vi "TX_basic.vi"() -> ()   [LabVIEW 2019]
uses:
  <vilib>/sound2/lvsound2.llb/Sound File Info (path).vi
  <vilib>/sound2/lvsound2.llb/Sound File Read Open.vi
  <vilib>/Analysis/2dsp.llb/Rational Resample (single channel, DBL).vi
  <vilib>/express/express analysis/Spectral/Block/exnSpectralBlock spectral measurements RMS poly.vi
  <vilib>/express/express analysis/Spectral/Block/exnSpectralBlock spectral measurements RMS DDT.vi
  <instrlib>/niUSRP/niUSRP Write Tx Data (CDB).vi
  <vilib>/sound2/lvsound2.llb/Sound File Read (DBL).vi
  <vilib>/express/express analysis/Spectral/XNode/ExpressSpectralMeasurementsBlockNode.xnode
  <vilib>/Analysis/NI_AALPro.lvlib
panel:
  out "Waveform Graph 2":dynamicdata(graph)
  in  "active antenna":string="TX1"
  out "error out":errorcluster
  out "coerced gain":dbl format="%#_6f"
  out "coerced carrier frequency":dbl=2400000000.0 format="%#_6p"
  out "coerced IQ rate":dbl=200000.0 format="%#_6p"
  in  "gain":dbl format="%#_6f"
  in  "carrier frequency":dbl=2400000000.0 format="%#_6p"
  in  "IQ rate":dbl=200000.0 format="%#_6p"
  in  "IP":refnum<k15>="192.168.10.2"
  in  "number of samples/ch (-1: all)":i32=10000
  out "Waveform Graph":waveform(dbl)(graph)
  in  "FM deviation(HZ)":dbl(slide) scale=0.0..100000.0
  out "XY Graph":cluster{dbl[], dbl[]}(graph)
  in  "stop":bool
  in  "path":path
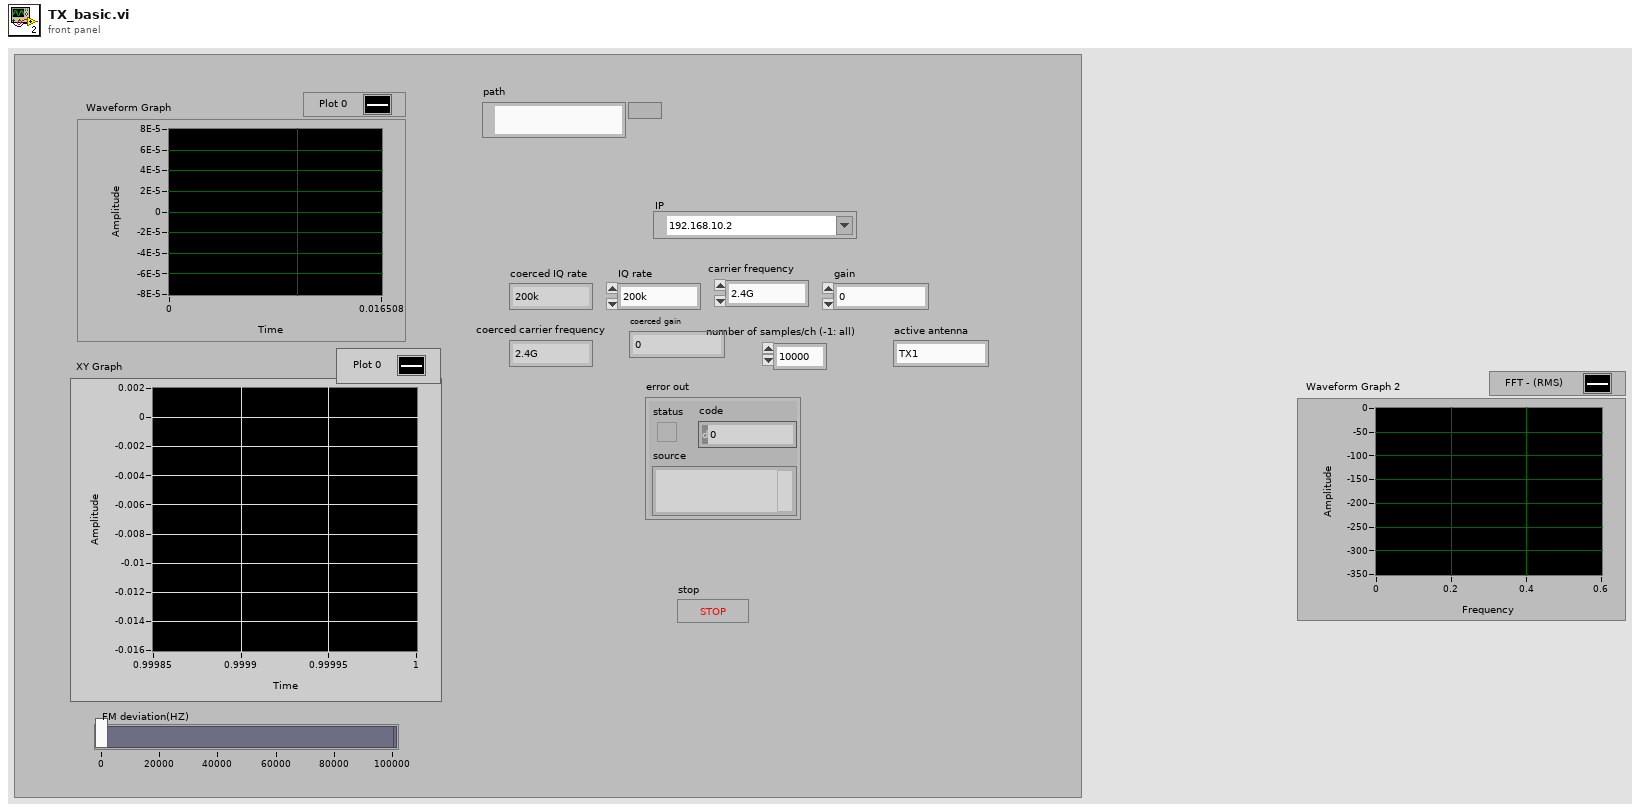
[diagram p1: front panel]
types:
  T1 = typedef "Sound Data Format.ctl" = cluster{"sample rate (S/s)":dbl, "number of channels":i32, "bits per sample":i32}
  T2 = typedef "Sound File Refnum.ctl" = refnum<file>
  T3 = cluster{"averaging mode":u16, "weighting mode":u16, "number of averages":u32}
  T4 = cluster{"dB On (F)":bool, "unwrap phase (F)":bool, "convert to degree (F)":bool}
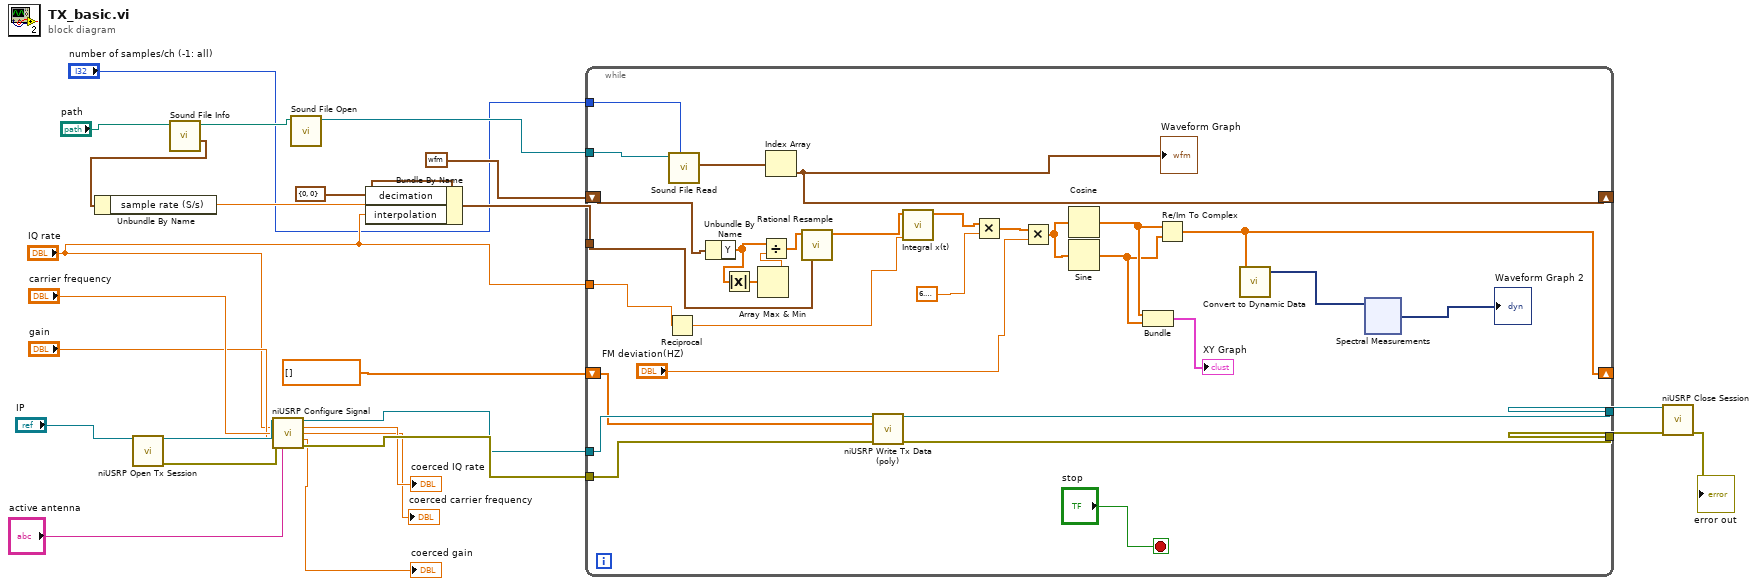
[diagram p0: block diagram]
diagram:
  n1 = call <instrlib>:"niUSRP Open Tx Session.vi"("device names"="IP") -> ("session handle out"=w21:refnum<k15>, "error out"=w20:errorcluster)  [unwired: 13 in]
  n2 = call-poly <vilib>:"Sound File Info.vi"("path"="path") -> ("sound format"=w8:T1, "path out"=w24:path)  [unwired: 7 in, 2 out]
  n3 = Unbundle By Name(w8) -> ("sample rate (S/s)"=w6:dbl)
  n4 = call <instrlib>:"niUSRP Configure Signal.vi"("session handle"=w21, "IQ rate"="IQ rate", "carrier frequency"="carrier frequency", "gain"="gain", "error in (no error)"=w20, "active antenna"="active antenna") -> ("session handle out"=w18:refnum<k15>, "coerced IQ rate"=→"coerced IQ rate":dbl, "coerced carrier frequency"=→"coerced carrier frequency":dbl, "coerced gain"=→"coerced gain":dbl, "error out"=w19:errorcluster)  [unwired: 5 in]
  n5 = call-poly <vilib>:"Sound File Open.vi"("path"=w24) -> ("sound file refnum"=w23:T2)  [unwired: 9 in, 1 out]
  n6 = Bundle By Name(cluster=cluster{"interpolation":i32, "decimation":i32} {"interpolation"=0, "decimation"=0} ("input cluster"), "decimation"=w6, "interpolation"="IQ rate") -> (w7:cluster{"interpolation":i32, "decimation":i32})
  n7 = while {
    tunnel: w23 -> [w55]
    shift-right: [w34] -> _
    shift-left: waveform(dbl) {"t0"=timestamp(0 s since 1904-01-01), "dt"=1.0, "Y"=[]} ("data") -> [w48]
    tunnel: "number of samples/ch (-1: all)" -> [w33]
    tunnel: w19 -> [w53]
    tunnel: w18 -> [w52]
    tunnel: "IQ rate" -> [w51]
    tunnel: [w50] -> w12
    tunnel: [w49] -> w11
    shift-right: [w31] -> _
    shift-left: cdb[] [] ("Array") -> [w40]
    tunnel: w7 -> [w39]
    stop <- "stop" stop-if-true
    n8 = Reciprocal(x=w51) -> (1/x=w46:dbl)
    n9 = call-poly <vilib>:"Sound File Read.vi"("number of samples/ch (-1: all)"=w33, "sound file refnum"=w55) -> ("data"=w54:waveform(dbl)[])  [unwired: 5 in, 4 out]
    n10 = Unbundle By Name(w48) -> ("Y"=w28:dbl[])
    n11 = Absolute Value(x=w28) -> (abs(x)=w29:dbl[])
    n12 = Array Max & Min(array=w29) -> (max value=w27:dbl)  [unwired: 3 out]
    n13 = Divide(x=w28, y=w27) -> (x/y=w26:dbl[])
    n14 = Index Array(array=w54) -> (element=w34:waveform(dbl))  [unwired: 1 in]
    "Waveform Graph" <- w34
    n15 = call-poly <vilib>:"Rational Resample.vi"("resample factor"=w39, "X"=w26) -> ("Y"=w47:dbl[])  [unwired: 7 in, 2 out]
    n16 = call-poly <instrlib>:"niUSRP Write Tx Data (poly).vi"("session handle"=w52, "data"=w40, "error in (no error)"=w53) -> ("session handle out"=w50:refnum<k15>, "error out"=w49:errorcluster)  [unwired: 11 in]
    n17 = call <vilib>:"Integral x(t).vi"("dt"=w46, "X"=w47) -> ("Integral X"=w45:dbl[])  [unwired: 8 in, 1 out]
    n18 = Multiply(x=w45, y=6.283185307179586) -> (x*y=w43:dbl[])
    n19 = Multiply(x=w43, y="FM deviation(HZ)") -> (x*y=w41:dbl[])
    n20 = Cosine(x=w41) -> (cos(x)=w38:dbl[])
    n21 = Sine(x=w41) -> (sin(x)=w37:dbl[])
    n22 = Bundle(w38, w37) -> (→"XY Graph":cluster{dbl[], dbl[]})  [unwired: 1 in]
    n23 = Re/Im To Complex(1:w37, 2:w38) -> (0:w31:cdb[])
    n24 = call "Convert to Dynamic Data"("Waveform"=w31) -> ("Dynamic Data Type"=w30:dynamicdata)  [unwired: 3 in]
    n25 = xnode ("Spectral Measurements")("信号"=w30) -> ("FFT - (RMS)"=→"Waveform Graph 2":dynamicdata)  [unwired: 1 in, 2 out]
  }
  n26 = call <instrlib>:"niUSRP Close Session.vi"("session handle"=w12, "error in (no error)"=w11) -> ("error out"=→"error out":errorcluster)  [unwired: 13 in]
